vi "LoadHexaSummary.vi"(7 "Machine":string, 10 "file path (dialog if empty)":path=path "C:/m300/HEXA/R141201634_20141222_141239.lot") -> (0 "error out":errorcluster)   [LabVIEW 2012]
uses:
  <vilib>/Utility/miscctls.llb/LVDateTimeRec.ctl
  <vilib>/addons/database/Auxilliary.llb/DB Tools Cursor Type.ctl
  <vilib>/addons/database/Connection.llb/DB Tools Open Connec (Path).vi
  <vilib>/addons/database/Connection.llb/Conn Execute.vi
  <vilib>/addons/database/Recordset.llb/Rec Fetch Integer Data (R).vi
  <vilib>/addons/database/Recordset.llb/Rec Destroy - Connection.vi
  <vilib>/addons/database/NI_Database_API.lvlib
panel:
  in  "Cluster 2":T1
  out "array":string[][](array[string])
  out "concatenated string":string
  in  "date time rec":T2
  in  "Cluster":T3
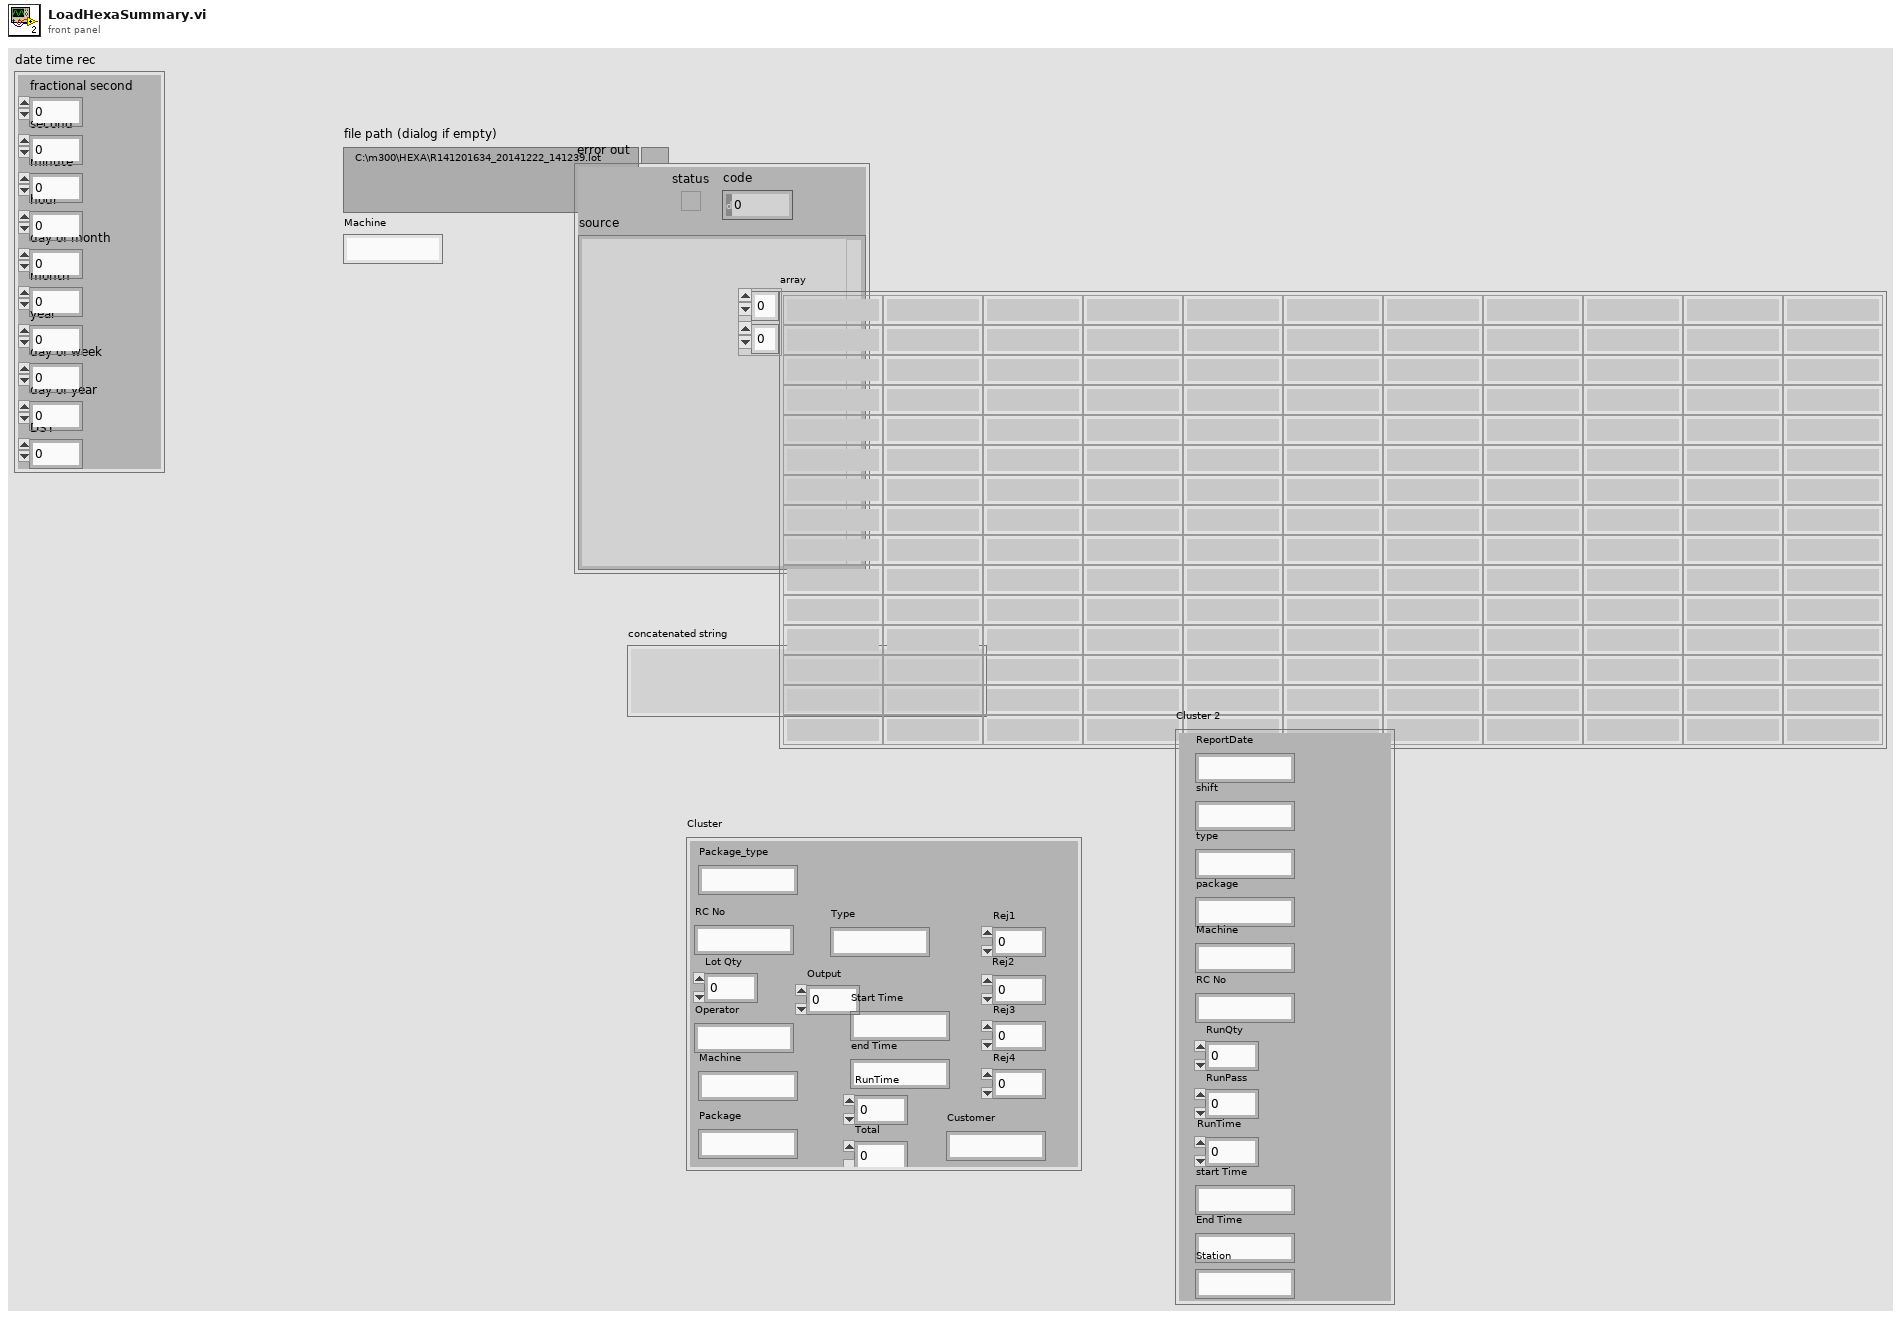
[diagram p1: front panel]
types:
  T1 = cluster{"ReportDate":string, "shift":string, "type":string, "package":string, "Machine":string, "RC No":string, "RunQty":dbl, "RunPass":dbl, "RunTime":dbl, "start Time":string, "End Time":string, "Station":string}
  T2 = typedef "LVDateTimeRec.ctl" = cluster{"fractional second":dbl, "second":i32, "minute":i32, "hour":i32, "day of month":i32, "month":i32, "year":i32, "day of week":i32, "day of year":i32, "DST":i32}
  T3 = cluster{"Package_type":string, "RC No":string, "Lot Qty":dbl, "Operator":string, "Machine":string, "Package":string, "Type":string, "Output":dbl, "Start Time":string, "end Time":string, "RunTime":dbl, "Total":dbl, "Rej1":dbl, "Rej2":dbl, "Rej3":dbl, "Rej4":dbl, "Customer":string}
  T4 = typedef "NI_Database_API.lvlib/DB Tools Cursor Type.ctl" = enum16{"forward-only", "keyset", "dynamic", "static"}
  T5 = typedef "NI_Database_API.lvlib/Conn ObjectReference.ctl" = refnum<k1>
  T6 = typedef "NI_Database_API.lvlib/Rec ObjectReference.ctl" = refnum<k1>
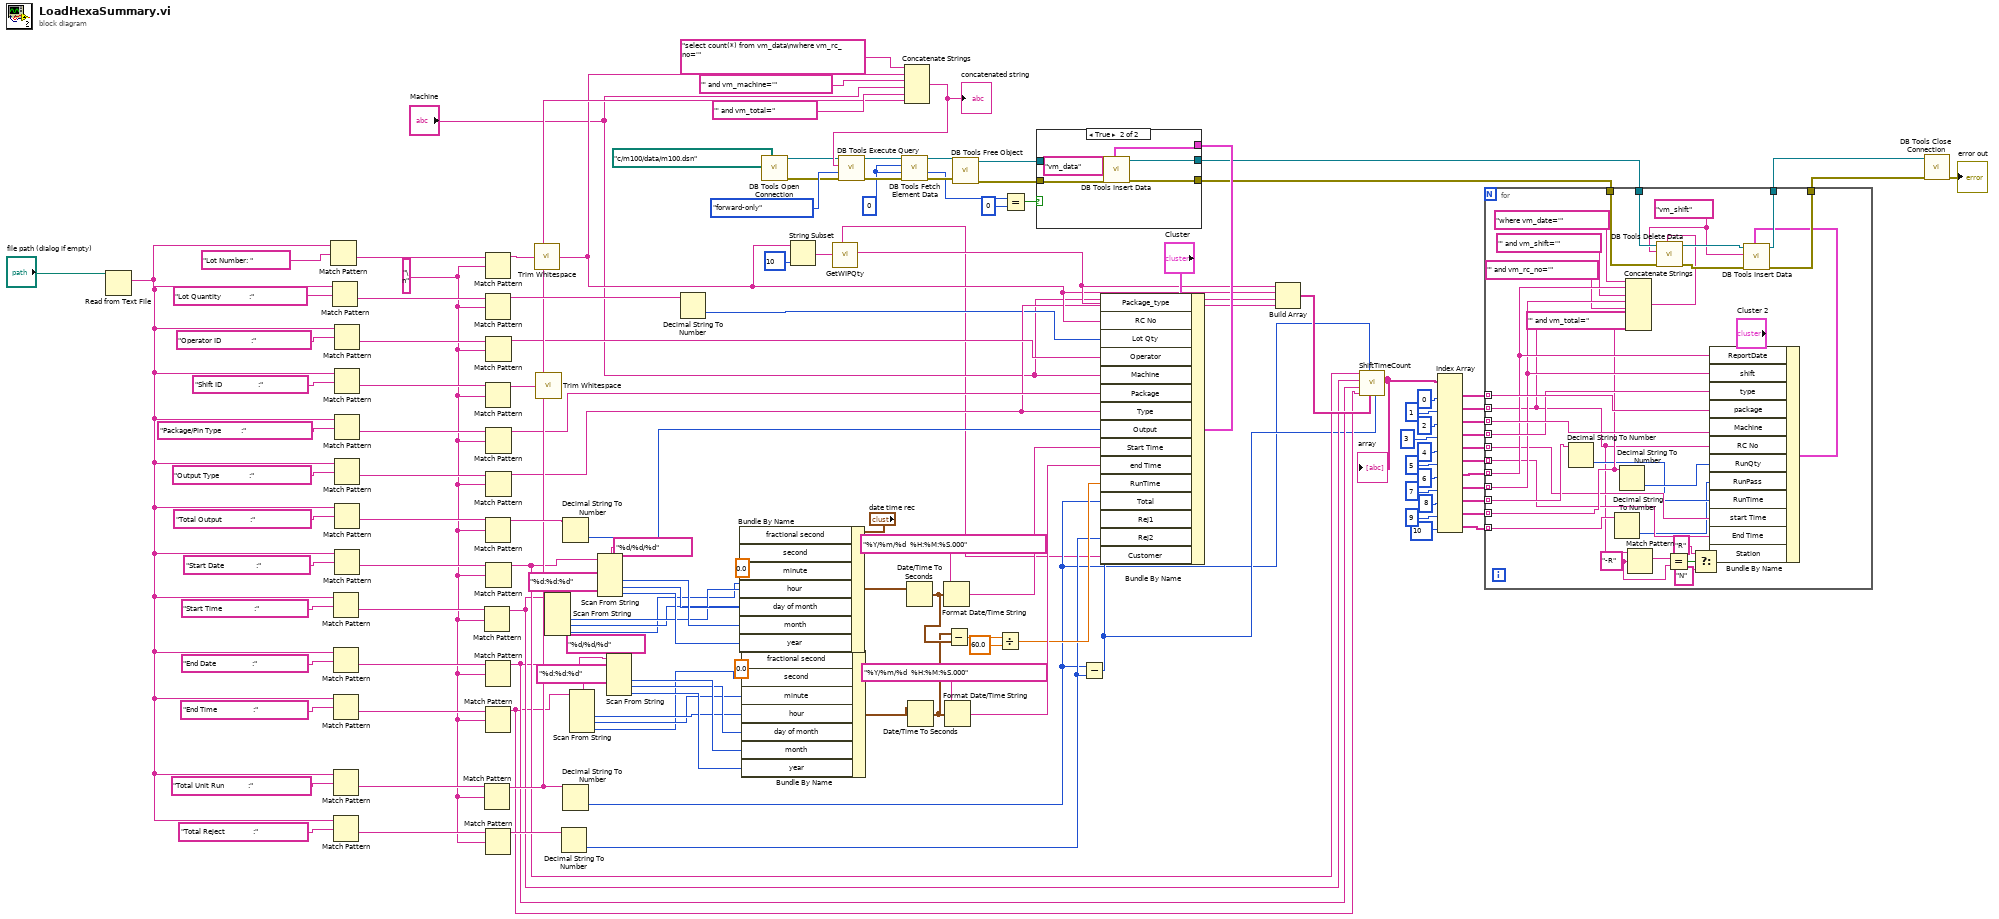
[diagram p0: block diagram]
diagram:
  w61 = 0
  w104 = "\n" ("regular expression")
  n1 = Read from Text File(file (use dialog)="file path (dialog if empty)") -> (text=w103:string)  [unwired: 3 in, 3 out]
  n2 = Match Pattern(string=w103, regular expression="Lot Number: ") -> (after substring=w129:string)  [unwired: 1 in, 3 out]
  n3 = Match Pattern(string=w103, regular expression="Lot Quantity              :") -> (after substring=w128:string)  [unwired: 1 in, 3 out]
  n4 = Match Pattern(string=w103, regular expression="Start Time                :") -> (after substring=w112:string)  [unwired: 1 in, 3 out]
  n5 = Match Pattern(string=w103, regular expression="End Date                  :") -> (after substring=w111:string)  [unwired: 1 in, 3 out]
  n6 = Match Pattern(string=w103, regular expression="End Time                  :") -> (after substring=w109:string)  [unwired: 1 in, 3 out]
  n7 = Match Pattern(string=w103, regular expression="Total Unit Run            :") -> (after substring=w106:string)  [unwired: 1 in, 3 out]
  n8 = Match Pattern(string=w103, regular expression="Total Reject              :") -> (after substring=w105:string)  [unwired: 1 in, 3 out]
  n9 = Match Pattern(string=w103, regular expression="Operator ID               :") -> (after substring=w125:string)  [unwired: 1 in, 3 out]
  n10 = Match Pattern(string=w103, regular expression="Shift ID                  :") -> (after substring=w122:string)  [unwired: 1 in, 3 out]
  n11 = Match Pattern(string=w103, regular expression="Package/Pin Type          :") -> (after substring=w121:string)  [unwired: 1 in, 3 out]
  n12 = Match Pattern(string=w103, regular expression="Output Type               :") -> (after substring=w119:string)  [unwired: 1 in, 3 out]
  n13 = Match Pattern(string=w103, regular expression="Total Output              :") -> (after substring=w116:string)  [unwired: 1 in, 3 out]
  n14 = Match Pattern(string=w103, regular expression="Start Date                :") -> (after substring=w115:string)  [unwired: 1 in, 3 out]
  n15 = Match Pattern(string=w112, regular expression=w104) -> (before substring=w34:string)  [unwired: 1 in, 3 out]
  n16 = Match Pattern(string=w106, regular expression=w104) -> (before substring=w47:string)  [unwired: 1 in, 3 out]
  n17 = Match Pattern(string=w129, regular expression=w104) -> (before substring=w54:string)  [unwired: 1 in, 3 out]
  n18 = Match Pattern(string=w128, regular expression=w104) -> (before substring=w127:string)  [unwired: 1 in, 3 out]
  n19 = Match Pattern(string=w122, regular expression=w104) -> (before substring=w53:string)  [unwired: 1 in, 3 out]
  n20 = Match Pattern(string=w116, regular expression=w104) -> (before substring=w102:string)  [unwired: 1 in, 3 out]
  n21 = Match Pattern(string=w111, regular expression=w104) -> (before substring=w33:string)  [unwired: 1 in, 3 out]
  n22 = Match Pattern(string=w109, regular expression=w104) -> (before substring=w32:string)  [unwired: 1 in, 3 out]
  n23 = Match Pattern(string=w105, regular expression=w104) -> (before substring=w72:string)  [unwired: 1 in, 3 out]
  n24 = Match Pattern(string=w125, regular expression=w104) -> (before substring=w41:string)  [unwired: 1 in, 3 out]
  n25 = Match Pattern(string=w121, regular expression=w104) -> (before substring=w46:string)  [unwired: 1 in, 3 out]
  n26 = Match Pattern(string=w119, regular expression=w104) -> (before substring=w40:string)  [unwired: 1 in, 3 out]
  n27 = Match Pattern(string=w115, regular expression=w104) -> (before substring=w35:string)  [unwired: 1 in, 3 out]
  n28 = call <vilib>:"Trim Whitespace.vi"("string"=w54) -> ("trimmed string"=w42:string)  [unwired: 1 in]
  n29 = call <vilib>:"Trim Whitespace.vi"("string"=w53) -> ()  [unwired: 1 in, 1 out]
  n30 = Scan From String(format string="%d:%d:%d", input string=w34) -> (output 1=w96:i32, output 2=w95:i32, output 3=w94:i32)  [unwired: 5 in, 3 out]
  n31 = Decimal String To Number(string=w72) -> (number=w70:i32)  [unwired: 2 in, 1 out]
  n32 = Decimal String To Number(string=w102) -> (number=w75:i32)  [unwired: 2 in, 1 out]
  n33 = Decimal String To Number(string=w47) -> (number=w2:i32)  [unwired: 2 in, 1 out]
  n34 = Scan From String(format string="%d:%d:%d", input string=w32) -> (output 1=w86:i32, output 2=w85:i32, output 3=w84:i32)  [unwired: 5 in, 3 out]
  n35 = Scan From String(format string="%d/%d/%d", input string=w35) -> (output 1=w100:i32, output 2=w99:i32, output 3=w98:i32)  [unwired: 5 in, 3 out]
  n36 = Scan From String(format string="%d/%d/%d", input string=w33) -> (output 1=w89:i32, output 2=w88:i32, output 3=w87:i32)  [unwired: 5 in, 3 out]
  n37 = Decimal String To Number(string=w127) -> (number=w37:i32)  [unwired: 2 in, 1 out]
  n38 = Bundle By Name(cluster="date time rec", "fractional second"=0.0, "second"=w94, "minute"=w95, "hour"=w96, "day of month"=w99, "month"=w100, "year"=w98) -> (w82:T2)
  n39 = Bundle By Name(cluster="date time rec", "fractional second"=0.0, "second"=w84, "minute"=w85, "hour"=w86, "day of month"=w88, "month"=w89, "year"=w87) -> (w79:T2)
  n40 = call-poly <vilib>:"DB Tools Open Connection.vi"("connection information"=path "c:/m100/data/m100.dsn") -> ("error out"=w50:errorcluster, "connection reference"=w51:T5)  [unwired: 7 in]
  n41 = String Subset(string=w42, length (rest)=10 ("length (rest)")) -> (substring=w44:string)  [unwired: 1 in]
  n42 = call "GetWIPQty.vi"("Lotno"=w44) -> ("Package"=w43:string, "CustomerID"=w1:string)  [unwired: 2 in, 7 out]
  n43 = Concatenate Strings("select count(*) from vm_data\nwhere vm_rc_no='" ("SQL query"), w42, "' and vm_machine='" ("string"), "Machine", "' and vm_total=" ("string"), w47) -> (w52:string)
  "concatenated string" <- w52
  n44 = call-poly <vilib>:"DB Tools Execute Query.vi"("error in (no error)"=w50, "cursor type"=DB_Tools_Cursor_Type."forward-only", "SQL query"=w52, "connection reference"=w51) -> ("error out"=w67:errorcluster, "recordset reference"=w69:T6)  [unwired: 4 in]
  n45 = call-poly <vilib>:"DB Tools Fetch Element Data.vi"("error in (no error)"=w67, "type"=w61, "column index"=w61, "recordset reference"=w69) -> ("error out"=w66:errorcluster, "data"=w60:i32, "recordset reference out"=w68:T6)  [unwired: 3 in]
  n46 = Date/Time To Seconds(2:w82) -> (0:w39:timestamp)  [unwired: 1 in]
  n47 = Date/Time To Seconds(2:w79) -> (0:w38:timestamp)  [unwired: 1 in]
  n48 = Format Date/Time String(time format string (%c)="%Y/%m/%d  %H:%M:%S.000", seconds (now)=w39) -> (date/time string=w74:string)  [unwired: 1 in]
  n49 = Format Date/Time String(time format string (%c)="%Y/%m/%d  %H:%M:%S.000", seconds (now)=w38) -> (date/time string=w73:string)  [unwired: 1 in]
  n50 = Subtract(x=w38, y=w39) -> (x-y=w78:dbl)
  n51 = call-poly <vilib>:"DB Tools Free Object.vi"("error in (no error)"=w66, "recordset reference"=w68) -> ("error out"=w56:errorcluster, "connection reference"=w57:T5)  [unwired: 8 in]
  n52 = Divide(x=w78, y=60.0) -> (x/y=w71:dbl)
  n53 = Equal?(x=w60, y=0) -> (x = y?=w58:bool)
  n54 = Subtract(x=w2, y=w70) -> (x-y=w3:i32)
  n55 = Bundle By Name(cluster="Cluster", "Package_type"=w43, "RC No"=w42, "Lot Qty"=w37, "Operator"=w41, "Machine"="Machine", "Package"=w46, "Type"=w40, "Output"=w75, "Start Time"=w74, "end Time"=w73, "RunTime"=w71, "Total"=w2, "Rej1"=w3, "Rej2"=w70, "Customer"=w1) -> (w55:T3)
  n56 = case shown="True" w58 {
    tunnel: w57 -> [w134 w140]
    tunnel: w56 -> [w133 w139]
    tunnel: [w134 w138] -> w9
    tunnel: [w133 w137] -> w8
    tunnel: w55 -> [_ w136]
    frame False {
    }
    frame True {
      n57 = call <vilib>:"DB Tools Insert Data.vi"("data"=w136, "error in (no error)"=w139, "table"="vm_data", "connection reference"=w140) -> ("error out"=w137:errorcluster, "connection reference out"=w138:T5)  [unwired: 6 in]
    }
  }
  n58 = Build Array(w43, w42, "Machine", w40) -> (w36:string[])
  n59 = call "ShiftTimeCount.vi"("PASS"=w3, "BasicData"=w36, "Qty"=w2, "EndTime 2"=w32, "date string"=w33, "BegTime"=w34, "BegDate"=w35) -> ("array"=w30:string[][])  [unwired: 4 in]
  "array" <- w30
  n60 = Index Array(array=w30, index (col) #1=0 ("disabled index (col)"), index (col) #2=1 ("index (col)"), index (col) #3=2 ("index (col)"), index (col) #4=3 ("index (col)"), index (col) #5=4 ("index (col)"), index (col) #6=5 ("index (col)"), index (col) #7=6 ("index (col)"), index (col) #8=7 ("index (col)"), index (col) #9=8 ("index (col)"), index (col) #10=9 ("index (col)"), index (col) #11=10 ("index (col)")) -> (element #1=w19:string[], element #2=w18:string[], element #3=w17:string[], element #4=w16:string[], element #5=w15:string[], element #6=w14:string[], element #7=w13:string[], element #8=w12:string[], element #9=w11:string[], element #10=w10:string[], element #11=w4:string[])  [unwired: 11 in]
  n61 = for {
    tunnel: w19 -> [w173] mode=indexing
    tunnel: w18 -> [w147] mode=indexing
    tunnel: w17 -> [w172] mode=indexing
    tunnel: w16 -> [w171] mode=indexing
    tunnel: w15 -> [w151] mode=indexing
    tunnel: w14 -> [w152] mode=indexing
    tunnel: w13 -> [w158] mode=indexing
    tunnel: w12 -> [w156] mode=indexing
    tunnel: w11 -> [w170] mode=indexing
    tunnel: w10 -> [w153] mode=indexing
    tunnel: w9 -> [w163]
    tunnel: w8 -> [w162]
    tunnel: [w168] -> w7
    tunnel: [w167] -> w6
    tunnel: w4 -> [w148] mode=indexing
    w145 = "-R" ("regular expression")
    w161 = "vm_shift" ("table")
    n62 = Decimal String To Number(string=w170) -> (number=w150:i32)  [unwired: 2 in, 1 out]
    n63 = Decimal String To Number(string=w148) -> (number=w149:i32)  [unwired: 2 in, 1 out]
    n64 = Decimal String To Number(string=w153) -> (number=w169:i32)  [unwired: 2 in, 1 out]
    n65 = Concatenate Strings("where vm_date='" ("string"), w158, "' and vm_shift='" ("string"), w156, "' and vm_rc_no='" ("string"), w147, "' and vm_total=" ("string"), w153) -> (w160:string)
    n66 = Match Pattern(string=w147, regular expression=w145) -> (match substring=w146:string)  [unwired: 1 in, 3 out]
    n67 = call <vilib>:"DB Tools Delete Data.vi"("condition"=w160, "error in (no error)"=w162, "table"=w161, "connection reference"=w163) -> ("error out"=w164:errorcluster, "connection reference out"=w165:T5)  [unwired: 6 in]
    n68 = Equal?(x=w146, y=w145) -> (x = y?=w144:bool)
    n69 = Select(t="R", s=w144, f="N") -> (s? t:f=w141:string)
    n70 = Bundle By Name(cluster="Cluster 2", "ReportDate"=w158, "shift"=w156, "type"=w171, "package"=w173, "Machine"=w172, "RC No"=w147, "RunQty"=w169, "RunPass"=w149, "RunTime"=w150, "start Time"=w151, "End Time"=w152, "Station"=w141) -> (w166:T1)
    n71 = call <vilib>:"DB Tools Insert Data.vi"("data"=w166, "error in (no error)"=w164, "table"=w161, "connection reference"=w165) -> ("error out"=w167:errorcluster, "connection reference out"=w168:T5)  [unwired: 6 in]
  }
  n72 = call <vilib>:"DB Tools Close Connection.vi"("error in (no error)"=w6, "connection reference"=w7) -> ("error out"=→"error out":errorcluster)  [unwired: 5 in]
